vi "unregister websocket.vi"(11 "parameters":variant) -> ()   [LabVIEW 2016, in "websocket upgrade handler.lvclass"]
uses:
  websocket upgrade handler.lvclass
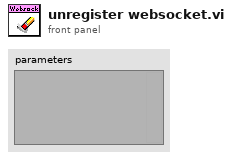
[diagram p1: front panel]
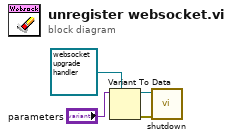
[diagram p0: block diagram]
diagram:
  n1 = Variant To Data(type=refnum<class "websocket upgrade handler.lvclass"> refnum ("websocket handler"), Variant="parameters") -> (data=w2:refnum<class "websocket upgrade handler.lvclass">, error out=w1:errorcluster)  [unwired: 1 in]
  n2 = call "shutdown.vi"("error in"=w1, "websocket handler in"=w2) -> ()  [unwired: 9 in, 1 out]
